vi "ReadMultiPoint.vi"(8 "error in (no error)":errorcluster, 11 "HP3458aDMM in":refnum<class "HP3458aDMM.lvclass">) -> (0 "error out":errorcluster, 3 "HP3458aDMM out":refnum<class "HP3458aDMM.lvclass">)   [LabVIEW 2014, in "SamplerPlugins.lvlib" / "HP3458aDMM.lvclass"]
uses:
  HP3458aDMM.lvclass
  NISTSamplerPluginsBaseClass/TypeDefs/MultiPointReadingParams.ctl
  NISTSamplerPluginsBaseClass/SamplerPluginsBase.lvclass
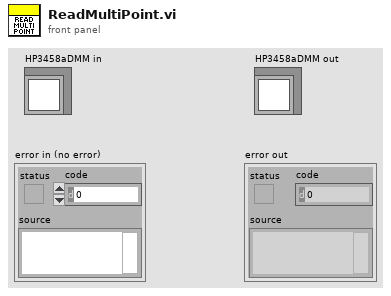
[diagram p1: front panel]
types:
  T1 = typedef "SamplerPlugins.lvlib/SamplerPluginsBase.lvclass/MultiPointReadingParams.ctl" = cluster{"dReadingArray":dbl[], "iActualPts":i32, "Timestamp":dbl}
  T2 = typedef "SamplerPlugins.lvlib/SamplerPluginsBase.lvclass/ReadMultiPointParams.ctl" = cluster{"iMaxTimeMilliseconds":i32, "iArraySize":i32}
  T3 = typedef "SamplerPlugins.lvlib/SamplerPluginsBase.lvclass/ConfigMultiPointParams.ctl" = cluster{"iTriggerCount":i32, "iSampleCount":i32, "eSampleClock":u16, "dSampleInterval":dbl}
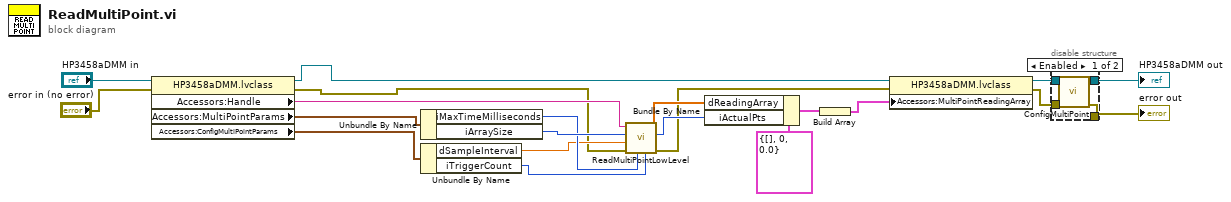
[diagram p0: block diagram]
diagram:
  n1 = property class="HP3458aDMM.lvclass"(reference="HP3458aDMM in", error in="error in (no error)") -> (reference out=w5:refnum<class "HP3458aDMM.lvclass">, error out=w6:errorcluster, "Accessors:Handle"=w19:string, "Accessors:MultiPointParams"=w15:T2, "Accessors:ConfigMultiPointParams"=w12:T3)
  n2 = Unbundle By Name(w15) -> ("iMaxTimeMilliseconds"=w13:i32, "iArraySize"=w14:i32)
  n3 = Unbundle By Name(w12) -> ("dSampleInterval"=w11:dbl, "iTriggerCount"=w9:i32)
  n4 = call "ReadMultiPointLowLevel.vi"("iTriggerCount"=w9, "iMaxTimeMilliseconds"=w13, "error in (no error)"=w6, "dSampleInterval"=w11, "iArraySize"=w14, "Handle"=w19) -> ("error out"=w10:errorcluster, "iActualPts"=w16:i32, "dReadingArray"=w17:dbl[])  [unwired: 3 in]
  n5 = Bundle By Name(cluster=T1 {"dReadingArray"=[], "iActualPts"=0, "Timestamp"=0.0} ("MultiPointReadingParams"), "dReadingArray"=w17, "iActualPts"=w16) -> (w8:T1)
  n6 = Build Array(w8) -> (w7:T1[])
  n7 = property class="HP3458aDMM.lvclass"(reference=w5, error in=w10, "Accessors:MultiPointReadingArray"=w7) -> (reference out=w4:refnum<class "HP3458aDMM.lvclass">, error out=w2:errorcluster)
  n8 = disable-structure shown="Enabled" {
    disable-tunnel: w4 -> [w25 w27]
    disable-tunnel: [w24 w27] -> w3
    disable-tunnel: w2 -> [w23 w26]
    disable-tunnel: [w22 w26] -> w1
    frame Enabled {
      n9 = call-dynamic "ConfigMultiPoint.vi"("error in (no error)"=w23, "HP3458aDMM in"=w25) -> ("error out"=w22:errorcluster, "HP3458aDMM out"=w24:refnum<class "HP3458aDMM.lvclass">)  [unwired: 8 in]
    }
    frame Disabled {
    }
  }
  "error out" <- w1
  "HP3458aDMM out" <- w3
